vi "configure.vi"(8 "error in (no error)":errorcluster, 9 "Value":i32, 10 "ILC":refnum<class "ILC.lvclass">, 11 "ConfigureILCCH0 in":refnum<class "ConfigureILCCH0Strategy.lvclass">) -> (0 "error out":errorcluster, 2 "ILC 2":refnum<class "ILC.lvclass">, 3 "ConfigureILCCH0 out":refnum<class "ConfigureILCCH0Strategy.lvclass">)   [LabVIEW 2015, in "ConfigureILCCH0Strategy.lvclass"]
uses:
  ConfigureILCCH0Strategy.lvclass
  <userlib>/Common/ILC/ILC/ILC.lvclass
  <userlib>/Common/ILC/ILC/ILC.lvclass/ILC.ctl
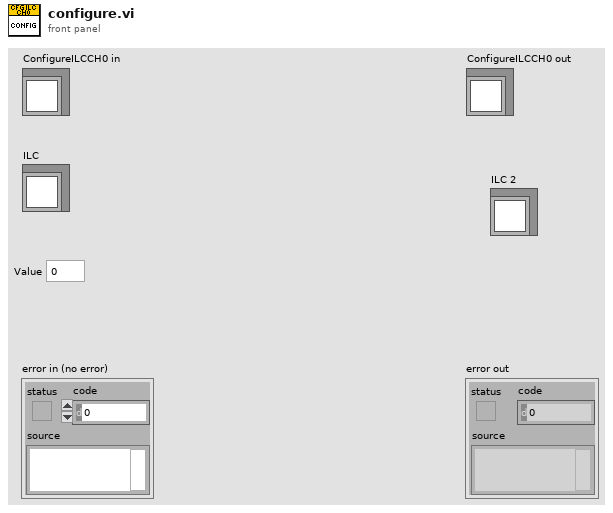
[diagram p1: front panel]
types:
  T1 = typedef "ILCCommon.lvlib/ILCTypedefs.lvlib/Outputs.ctl" = cluster{"Step & Direction":i16, "Blower RPM":u8, "PWM (SSR)":u8, "Ch1":u16, "Ch2":u16, "Ch3":u16, "Ch4":u16}
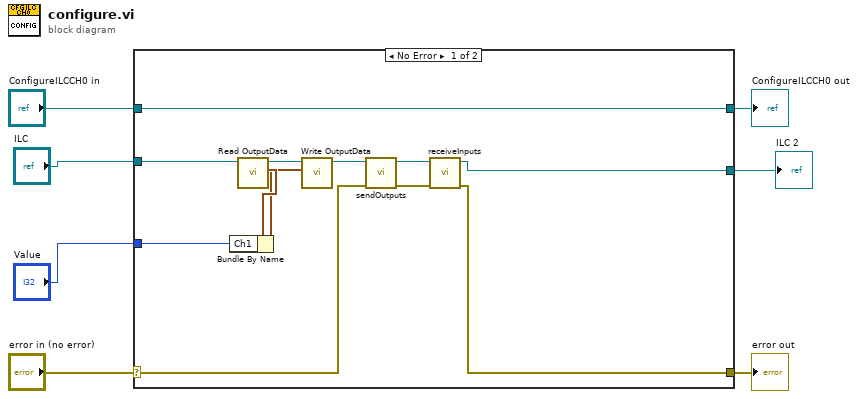
[diagram p0: block diagram]
diagram:
  n1 = case shown="No Error" "error in (no error)" {
    selector: "error in (no error)" -> [w11 w22]
    tunnel: [w9 w22] -> w6
    tunnel: [w19 w21] -> w4
    tunnel: "ConfigureILCCH0 in" -> [w19 w21]
    tunnel: "ILC" -> [w18 w20]
    tunnel: "Value" -> [w16 _]
    tunnel: [w8 w20] -> w1
    frame No Error {
      n2 = call <userlib>:"Read OutputData.vi"("ILC in"=w18) -> ("OutputData"=w17:T1, "ILC out"=w14:refnum<class "ILC.lvclass">)  [unwired: 9 in]
      n3 = Bundle By Name(cluster=w17, "Ch1"=w16) -> (w15:T1)
      n4 = call <userlib>:"Write OutputData.vi"("OutputData"=w15, "ILC in"=w14) -> ("ILC out"=w13:refnum<class "ILC.lvclass">)  [unwired: 9 in]
      n5 = call <userlib>:"sendOutputs.vi"("error in (no error)"=w11, "ILC in"=w13) -> ("error out"=w10:errorcluster, "ILC out"=w12:refnum<class "ILC.lvclass">)  [unwired: 8 in]
      n6 = call <userlib>:"receiveInputs.vi"("error in (no error)"=w10, "ILC in"=w12) -> ("error out"=w9:errorcluster, "ILC out"=w8:refnum<class "ILC.lvclass">)  [unwired: 6 in, 2 out]
    }
    frame Error {
    }
  }
  "error out" <- w6
  "ConfigureILCCH0 out" <- w4
  "ILC 2" <- w1
